vi "Test Assertion.vi"(8 "error in (no error)":errorcluster, 11 "Step":T1={"Type"=enum."Mouse Move", "X"=0, "Y"=0, "Delay"=0, "Key"=65, "Repeat"=0, "RClick?"=FALSE, "App/Window Name"="", "Notes"="", "Assertion Type"=enum."Control Position", "Control Name"="", "Disabled"=enum."Enabled", "Visible"=enum."Visible", "Left"=0, "Top"=0, "Width"=0, "Height"=0, "Expected Image"={"image type"=0, "image depth"=0, "image"=[], "mask"=[], "colors"=[], "Rectangle"={"left"=0, "top"=0, "right"=0, "bottom"=0}}}) -> (0 "error out":errorcluster, 2 "Actual Value":variant, 3 "Pass?":bool)   [LabVIEW 2020, in "MacroAssert.lvlib"]
uses:
  MacroAssert.lvlib
  CTLs/Step Type V3.ctl
  CTLs/Assertion Type.ctl
  <vilib>/picture/picture.llb/imagedata.ctl
  CTLs/Step V3.ctl
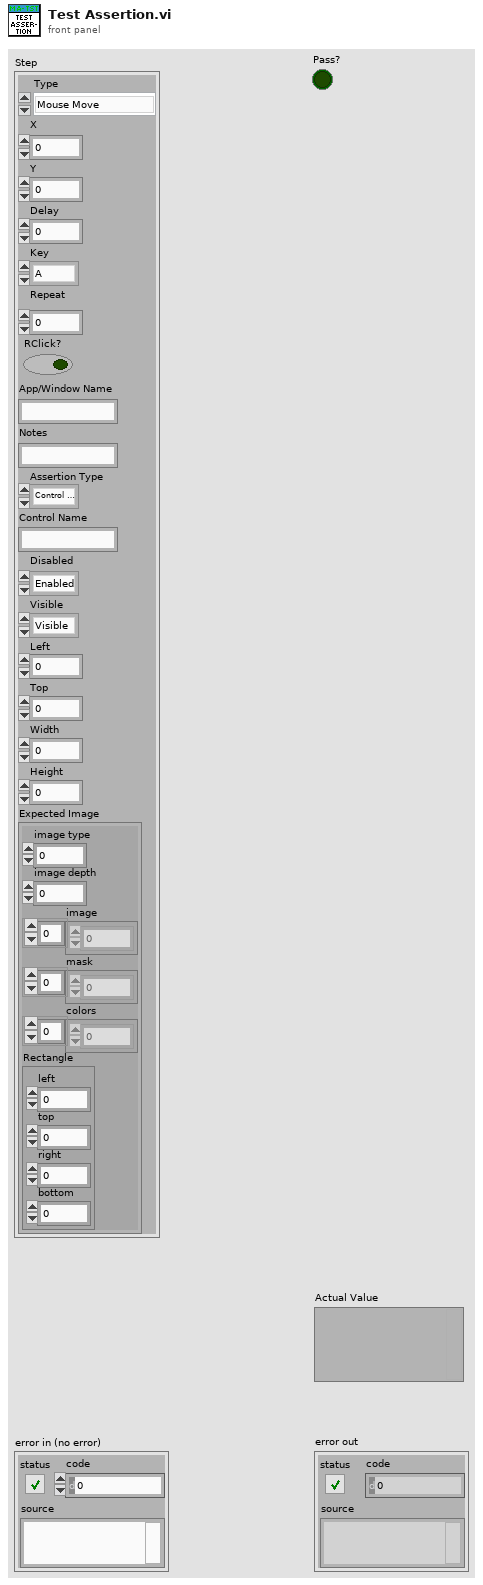
[diagram p1: front panel]
types:
  T1 = typedef "MacroAssert.lvlib/Step V3.ctl" = cluster{"Type":T2, "X":i32, "Y":i32, "Delay":i32, "Key":u8, "Repeat":i32, "RClick?":bool, "App/Window Name":string, "Notes":string, "Assertion Type":T3, "Control Name":string, "Disabled":enum8{"Enabled", "Disabled", "Disabled and Grayed Out"}, "Visible":enum16{"Visible", "Not Visible"}, "Left":i16, "Top":i16, "Width":i16, "Height":i16, "Expected Image":T4}
  T2 = typedef "MacroAssert.lvlib/Step Type V3.ctl" = enum16{"Mouse Move", "Mouse Click", "Key Press", "Wait", "Mouse Down", "Mouse Up", "Key Down", "Key Up", "Test Assertion", "Run Application", "Maximize Window", "Restore Window", "Minimize Window", "Close Window", "Bring Window to Front", "Send Window to Back"}
  T3 = typedef "MacroAssert.lvlib/Assertion Type.ctl" = enum16{"Control Position", "Control Visible", "Control Disabled", "Control Image"}
  T4 = typedef "imagedata.ctl" = cluster{"image type":i32, "image depth":i32, "image":u8[], "mask":u8[], "colors":u32[], "Rectangle":cluster{"left":i16, "top":i16, "right":i16, "bottom":i16}}
  T5 = enum8{"Enabled", "Disabled", "Disabled and Grayed Out"}
  T6 = cluster{"left":i16, "top":i16, "right":i16, "bottom":i16}
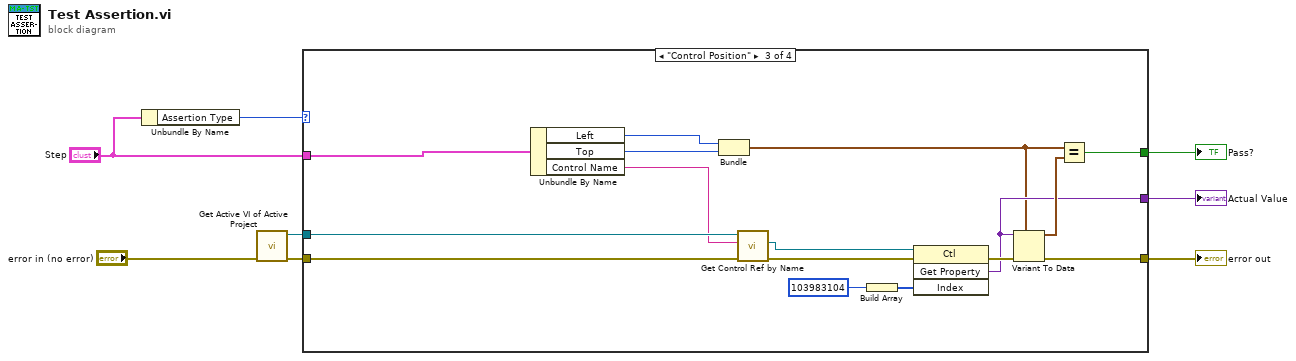
[diagram p0: block diagram]
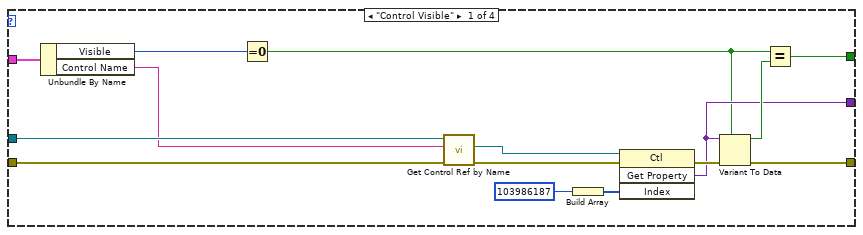
[diagram p2: hidden frame]
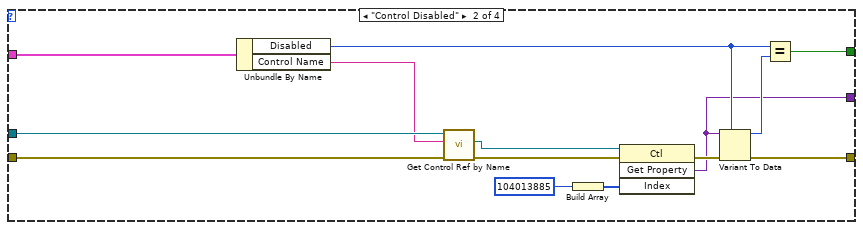
[diagram p3: hidden frame]
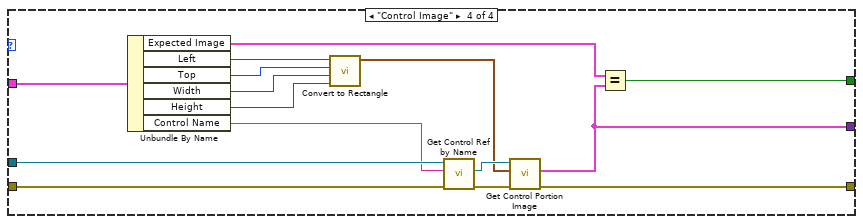
[diagram p4: hidden frame]
diagram:
  n1 = Unbundle By Name("Step") -> ("Assertion Type"=w2:T3)
  n2 = call "Get Active VI of Active Project.vi"("error in (no error)"="error in (no error)") -> ("error out"=w5:errorcluster, "Active VI Ref"=w4:refnum<vi>)  [unwired: 9 in]
  n3 = case shown="\"Control Position\"" w2 {
    tunnel: [w22 w36 w52 w61] -> w8
    tunnel: "Step" -> [w12 w24 w41 w66]
    tunnel: [w17 w31 w47 w67] -> w7
    tunnel: w5 -> [w20 w34 w50 w68]
    tunnel: w4 -> [w15 w27 w44 w64]
    tunnel: [w13 w25 w42 w60] -> w3
    frame "Control Visible" {
      n4 = Unbundle By Name(w12) -> ("Visible"=w10:enum16{"Visible", "Not Visible"}, "Control Name"=w11:string)
      n5 = Equal To 0?(x=w10) -> (x = 0?=w9:bool)
      n6 = call "Get Control Ref by Name.vi"("error in (no error)"=w20, "Name"=w11, "VI Ref"=w15) -> ("error out"=w21:errorcluster, "Ctl Ref"=w14:refnum<vi>)  [unwired: 6 in, 1 out]
      n7 = Build Array(103986187) -> (w18:i32[])
      n8 = invoke class="Ctl" method="Get Property"(reference=w14, error in=w21, "Index"=w18) -> (error out=w23:errorcluster, "GetProperty"=w13:variant)  [unwired: 1 in, 2 out]
      n9 = Variant To Data(error in=w23, type=w9, Variant=w13) -> (data=w16:bool, error out=w22:errorcluster)
      n10 = Equal?(x=w9, y=w16) -> (x = y?=w17:bool)
    }
    frame "Control Disabled" {
      n11 = Unbundle By Name(w24) -> ("Disabled"=w28:T5, "Control Name"=w26:string)
      n12 = call "Get Control Ref by Name.vi"("error in (no error)"=w34, "Name"=w26, "VI Ref"=w27) -> ("error out"=w35:errorcluster, "Ctl Ref"=w29:refnum<vi>)  [unwired: 6 in, 1 out]
      n13 = Build Array(104013885) -> (w32:i32[])
      n14 = invoke class="Ctl" method="Get Property"(reference=w29, error in=w35, "Index"=w32) -> (error out=w37:errorcluster, "GetProperty"=w25:variant)  [unwired: 1 in, 2 out]
      n15 = Variant To Data(error in=w37, type=w28, Variant=w25) -> (data=w30:T5, error out=w36:errorcluster)
      n16 = Equal?(x=w28, y=w30) -> (x = y?=w31:bool)
    }
    frame "Control Position" {
      n17 = Unbundle By Name(w41) -> ("Left"=w39:i16, "Top"=w40:i16, "Control Name"=w43:string)
      n18 = Bundle("Left"=w39, "Top"=w40) -> (w38:cluster{"Left":i16, "Top":i16})  [unwired: 1 in]
      n19 = call "Get Control Ref by Name.vi"("error in (no error)"=w50, "Name"=w43, "VI Ref"=w44) -> ("error out"=w51:errorcluster, "Ctl Ref"=w45:refnum<vi>)  [unwired: 6 in, 1 out]
      n20 = Build Array(103983104) -> (w48:i32[])
      n21 = invoke class="Ctl" method="Get Property"(reference=w45, error in=w51, "Index"=w48) -> (error out=w53:errorcluster, "GetProperty"=w42:variant)  [unwired: 1 in, 2 out]
      n22 = Variant To Data(error in=w53, type=w38, Variant=w42) -> (data=w46:cluster{"Left":i16, "Top":i16}, error out=w52:errorcluster)
      n23 = Equal?(x=w38, y=w46) -> (x = y?=w47:bool)
    }
    frame "Control Image" {
      n24 = Unbundle By Name(w66) -> ("Expected Image"=w59:T4, "Left"=w58:i16, "Top"=w57:i16, "Width"=w56:i16, "Height"=w55:i16, "Control Name"=w63:string)
      n25 = call "Convert to Rectangle.vi"("Height"=w55, "Width"=w56, "Top"=w57, "Left"=w58) -> ("Rectangle"=w54:T6)  [unwired: 7 in]
      n26 = call "Get Control Ref by Name.vi"("error in (no error)"=w68, "Name"=w63, "VI Ref"=w64) -> ("error out"=w62:errorcluster, "Ctl Ref"=w65:refnum<vi>)  [unwired: 6 in, 1 out]
      n27 = call "Get Control Portion Image.vi"("error in (no error)"=w62, "subset rect"=w54, "Ctl Ref"=w65) -> ("error out"=w61:errorcluster, "Ctl Portion Image Data"=w60:T4)  [unwired: 5 in, 2 out]
      n28 = Equal?(x=w59, y=w60) -> (x = y?=w67:bool)
    }
  }
  "error out" <- w8
  "Pass?" <- w7
  "Actual Value" <- w3
